vi "GV scan galvo delay.vi"() -> ()   [LabVIEW 2017]
panel:
  in  "ScanGalvoDelay_tick":u16
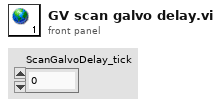
[diagram p1: front panel]
diagram:
